vi "listfiles.vi"(8 "Error In":errorcluster) -> (0 "error out":errorcluster)   [LabVIEW 2014, in "LabVIEW Universal Transcriptor SD Card Library.lvlib"]
uses:
  LabVIEW Universal Transcriptor SD Card Library.lvlib
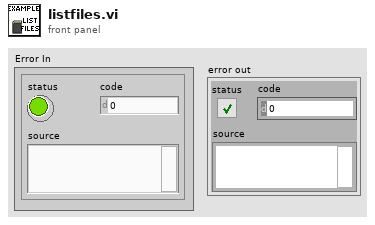
[diagram p1: front panel]
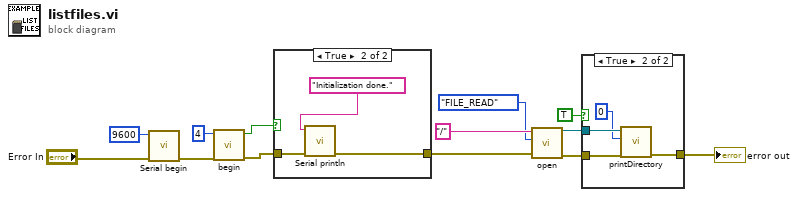
[diagram p0: block diagram]
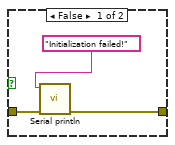
[diagram p3: hidden frame]
diagram:
  n1 = call <vilib>:"Serial begin.vi"("Error In"="Error In", "speed (Bd)"=9600) -> ("Error Out"=w12:errorcluster)  [unwired: 9 in]
  n2 = call "begin.vi"("Error In"=w12, "CS pin (optional)"=u8 4) -> ("Error Out"=w9:errorcluster, "success?"=w8:bool)  [unwired: 8 in]
  n3 = case shown="True" w8 {
    tunnel: w9 -> [w15 w18]
    tunnel: [w14 w17] -> w7
    frame False {
      n4 = call <vilib>:"Serial println.vi"("Error In"=w15, "string in"="Initialization failed!" ("filepath")) -> ("Error Out"=w14:errorcluster)  [unwired: 9 in]
    }
    frame True {
      n5 = call <vilib>:"Serial println.vi"("Error In"=w18, "string in"="Initialization done." ("filepath")) -> ("Error Out"=w17:errorcluster)  [unwired: 9 in]
    }
  }
  n6 = call "open.vi"("Error In"=w7, "mode"=enum16{"FILE_READ", "FILE_WRITE"}."FILE_READ", "filepath"="/") -> ("Error Out"=w4:errorcluster, "File out"=w3:refnum<class "File.lvclass">)  [unwired: 7 in]
  n7 = case shown="True" TRUE {
    tunnel: w4 -> [w20 w24]
    tunnel: w3 -> [_ w23]
    tunnel: [w20 w21] -> w2
    frame False {
    }
    frame True {
      n8 = call "printDirectory.vi"("Error In"=w24, "nested level"=u8 0, "file"=w23) -> ("Error Out"=w21:errorcluster)  [unwired: 8 in]
    }
  }
  "error out" <- w2
